vi "sub_UI_ref2.vi"(7 "cmd":T2, 11 "UI ctl2 in":T1) -> (3 "UI ctl2 out":T1)   [LabVIEW 2016]
uses:
  ctl/UI_cmd-ctl.ctl
  ctl/UI_ctl2.ctl
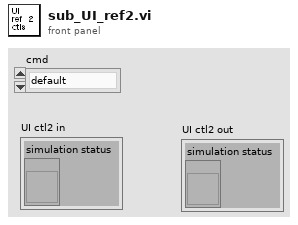
[diagram p1: front panel]
types:
  T1 = typedef "UI_ctl2.ctl" = cluster{"simulation status":refnum<vi>}
  T2 = typedef "UI_cmd-ctl.ctl" = enum16{"default", "create", "read"}
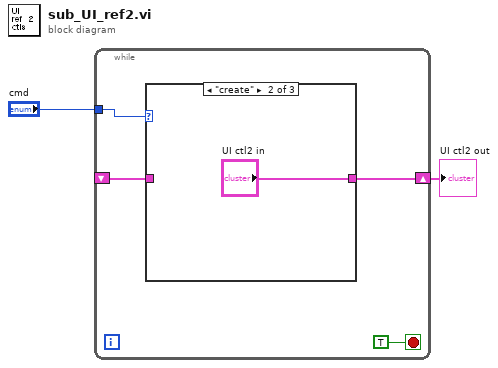
[diagram p0: block diagram]
diagram:
  n1 = while {
    tunnel: "cmd" -> [w6]
    shift-right: [w4] -> w1
    shift-left: _ -> [w3]
    stop <- TRUE stop-if-true
    n2 = case shown="\"create\"" w6 {
      tunnel: [w7 "UI ctl2 in" w9] -> w4
      tunnel: w3 -> [w7 _ w9]
      frame "default", Default {
      }
      frame "create" {
      }
      frame "read" {
      }
    }
  }
  "UI ctl2 out" <- w1
